vi "Serial Numberv.vi"(8 "error in":errorcluster, 10 "Serial No":cluster{"Serial Number":T1}, 11 "Read Write":enum16{"Read", "Write"}(ring)=enum."Write") -> (0 "error out":errorcluster, 2 "Serial No":cluster{"Serial Number":T1})   [LabVIEW 2024]
uses:
  <vilib>/Utility/config.llb/NI_LVConfig.lvlib
  Control 2.ctl
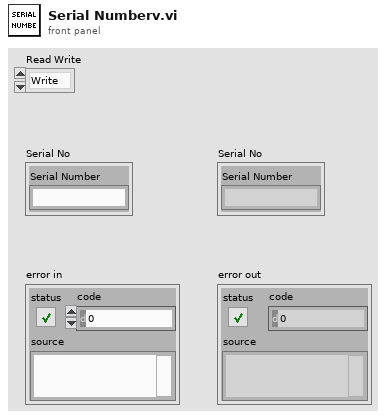
[diagram p1: front panel]
types:
  T1 = typedef "Control 2.ctl" = string
  T2 = typedef "File Paths.ctl" = cluster{"Log":path, "Report":path, "Error Info":path, "Event log":path, "Configuration":path, "Database":path, "Test Statistics":path, "User Accounts":path, "Video Folder":path, "Crimping Report":path}
  T3 = typedef "NI_LVConfig.lvlib/Config Data RefNum.ctl" = refnum<k1>
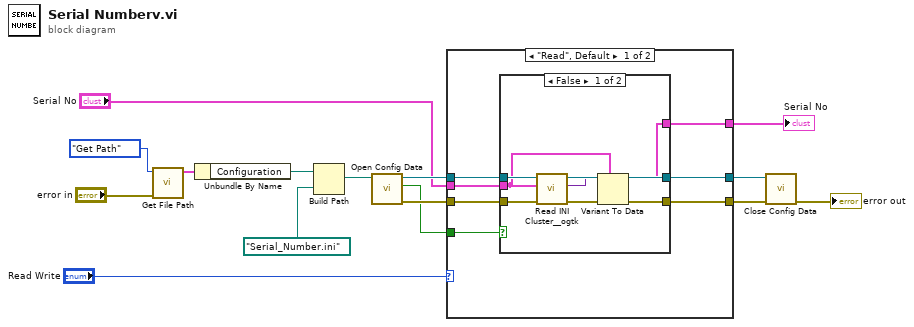
[diagram p0: block diagram]
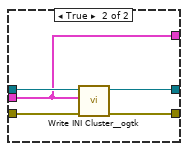
[diagram p2: hidden frame]
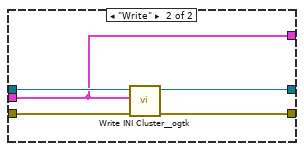
[diagram p3: hidden frame]
diagram:
  n1 = call "Get File Path.vi"("error in (no error)"="error in", "Action?"=enum16{"Initialize", "Get Path"}."Get Path") -> ("File Paths"=w15:T2)  [unwired: 8 in, 1 out]
  n2 = Unbundle By Name(w15) -> ("Configuration"=w13:path)
  n3 = Build Path(base path=w13, name or relative path=path "Serial_Number.ini") -> (appended path=w11:path)
  n4 = call <vilib>:"Open Config Data.vi"("configuration file path"=w11) -> ("error out"=w7:errorcluster, "file created?"=w5:bool, "refnum"=w10:T3)  [unwired: 8 in]
  n5 = case shown="\"Read\", Default" "Read Write" {
    tunnel: w10 -> [w22 w40]
    tunnel: [w21 w38] -> w9
    tunnel: "Serial No" -> [w20 w36]
    tunnel: w7 -> [w19 w39]
    tunnel: [w18 w37] -> w6
    tunnel: w5 -> [w17 _]
    tunnel: [w16 w36] -> w4
    frame "Read", Default {
      n6 = case shown="False" w17 {
        tunnel: w22 -> [w30 w35]
        tunnel: [w29 w33] -> w21
        tunnel: w20 -> [w24 w31]
        tunnel: w19 -> [w28 w34]
        tunnel: [w26 w32] -> w18
        tunnel: [w23 w31] -> w16
        frame False {
          n7 = call <userlib>:"Read INI Cluster__ogtk.vi"("error in (no error)"=w28, "INI Fomatted Cluster Type"=w24, "refnum"=w30) -> ("error out"=w27:errorcluster, "INI Fomatted Cluster"=w25:variant, "dup refnum"=w29:T3)  [unwired: 4 in, 2 out]
          n8 = Variant To Data(error in=w27, type=w24, Variant=w25) -> (data=w23:cluster{"Serial Number":T1}, error out=w26:errorcluster)
        }
        frame True {
          n9 = call <userlib>:"Write INI Cluster__ogtk.vi"("error in (no error)"=w34, "INI Fomatted Cluster"=w31, "refnum"=w35) -> ("error out"=w32:errorcluster, "dup refnum"=w33:T3)  [unwired: 7 in]
        }
      }
    }
    frame "Write" {
      n10 = call <userlib>:"Write INI Cluster__ogtk.vi"("error in (no error)"=w39, "INI Fomatted Cluster"=w36, "refnum"=w40) -> ("error out"=w37:errorcluster, "dup refnum"=w38:T3)  [unwired: 7 in]
    }
  }
  "Serial No" <- w4
  n11 = call <vilib>:"Close Config Data.vi"("error in (no error)"=w6, "refnum"=w9) -> ("error out"=→"error out":errorcluster)  [unwired: 8 in, 1 out]
